vi "Get Output Power.vi"(7 "VSEC":dbl, 8 "Position":i32, 9 "Number of Strings":i32, 10 "Test Voltage":string, 11 "Efficiency Test":refnum<class "Efficiency Test.lvclass">) -> (3 "Power Out":dbl)   [LabVIEW 2015, in "Efficiency Test.lvclass"]
uses:
  Efficiency Test.lvclass
  <vilib>/Cree, Inc/Cree Test Framework/Core Launcher/Core Manager Methods -- Enum.ctl
  <vilib>/Cree, Inc/Cree Test Framework/Classes/Variable Engine/Class/Variable Engine.lvclass
  <vilib>/Cree, Inc/Cree Test Framework/Core Launcher/Core Launcher.lvlib
  Test Class/Test Class.lvclass
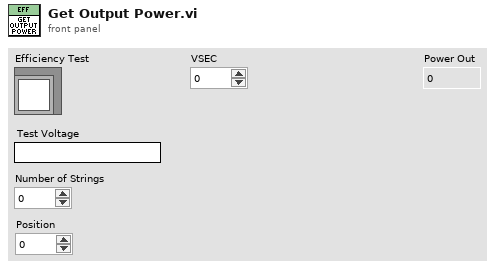
[diagram p1: front panel]
types:
  T1 = typedef "Core Launcher.lvlib/Core Manager Methods -- Enum.ctl" = enum16{"Spawn Objects", "Get Objects", "Destroy Objects"}
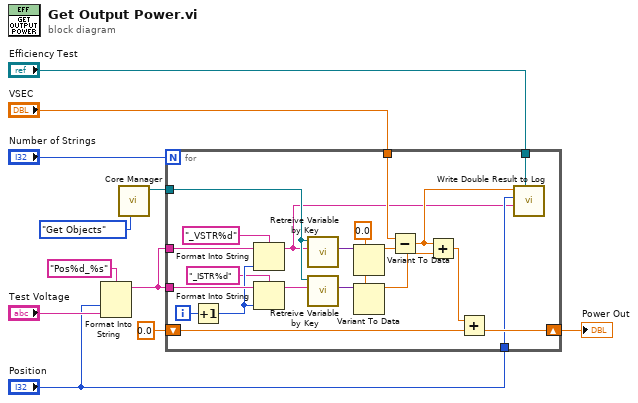
[diagram p0: block diagram]
diagram:
  n1 = Format Into String(format string="Pos%d_%s", "Position", "Test Voltage") -> (resulting string=w4:string)  [unwired: 2 in, 1 out]
  n2 = call <vilib>:"Core Manager.vi"("Method"=Core_Manager_Methods_--_Enum."Get Objects") -> ("Variable Engine"=w6:refnum<class "Variable Engine.lvclass">)  [unwired: 6 in, 4 out]
  n3 = for {
    N: "Number of Strings" -> [_]
    tunnel: w4 -> [w20]
    tunnel: w4 -> [w19]
    tunnel: "VSEC" -> [w30]
    shift-right: [w22] -> w11
    shift-left: 0.0 ("data") -> [w23]
    tunnel: w6 -> [w16]
    tunnel: "Position" -> [w13]
    tunnel: "Efficiency Test" -> [w15]
    i -> [w32]
    w26 = 0.0
    n4 = Increment(x=w32) -> (x+1=w18:i32)
    n5 = Format Into String(format string="_VSTR%d" ("string"), initial string=w20, w18) -> (resulting string=w12:string)  [unwired: 1 in, 1 out]
    n6 = Format Into String(format string="_ISTR%d" ("string"), initial string=w19, w18) -> (resulting string=w29:string)  [unwired: 1 in, 1 out]
    n7 = call <vilib>:"Retreive Variable by Key.vi"("Key"=w12, "Acrobat Template in"=w16) -> ("Value"=w28:variant)  [unwired: 7 in, 2 out]
    n8 = call <vilib>:"Retreive Variable by Key.vi"("Key"=w29, "Acrobat Template in"=w16) -> ("Value"=w27:variant)  [unwired: 7 in, 2 out]
    n9 = Variant To Data(type=w26, Variant=w28) -> (data=w25:dbl)  [unwired: 1 in, 1 out]
    n10 = Variant To Data(type=w26, Variant=w27) -> (data=w24:dbl)  [unwired: 1 in, 1 out]
    n11 = Subtract(x=w30, y=w25) -> (x-y=w14:dbl)
    n12 = Add(x=w14, y=w24) -> (x+y=w21:dbl)
    n13 = Add(x=w21, y=w23) -> (x+y=w22:dbl)
    n14 = call "Write Double Result to Log.vi"("Test Class in"=w15, "Label"=w12, "Position"=w13, "Value"=w14) -> ()  [unwired: 7 in, 1 out]
  }
  "Power Out" <- w11
